vi "openDevice.vi"(8 "error in (no error)":errorcluster, 10 "deviceName":string, 11 "AtomChipHWC in":refnum<class "AtomChipHWC.lvclass">) -> (0 "error out":errorcluster, 3 "AtomChipHWC out":refnum<class "AtomChipHWC.lvclass">)   [LabVIEW 2009, in "Hardware.lvlib" / "HWControllers.lvlib" / "AtomChipHWC.lvclass"]
doc: "Opens a device."
uses:
  AtomChipHWC.lvclass
  IntegrationManagement/CameraManager.lvclass
  AtomChipHWC.lvclass/AtomChipHWC.ctl
  HWController.lvclass
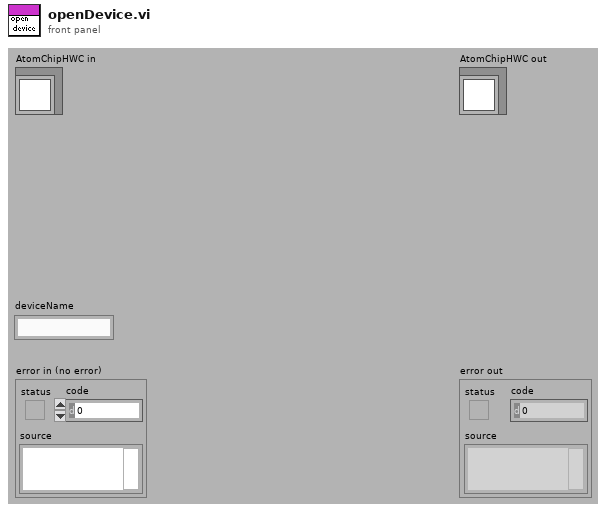
[diagram p1: front panel]
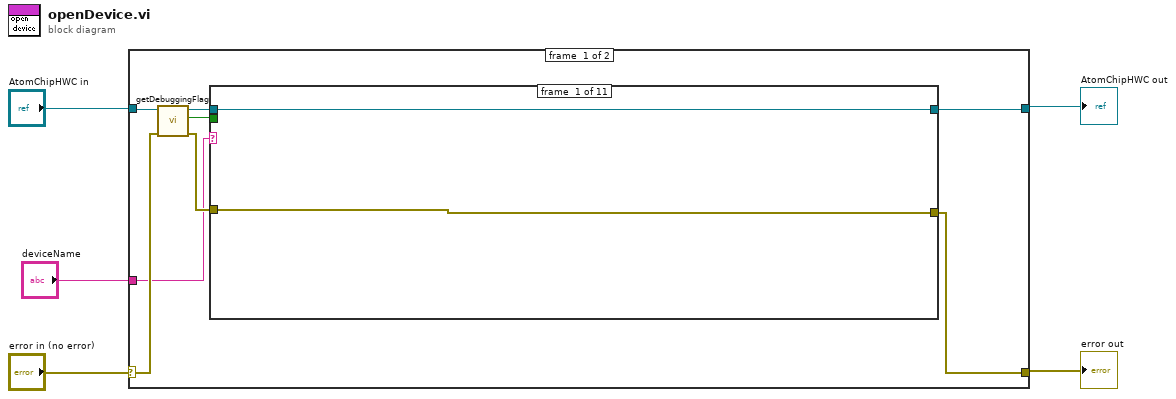
[diagram p0: block diagram]
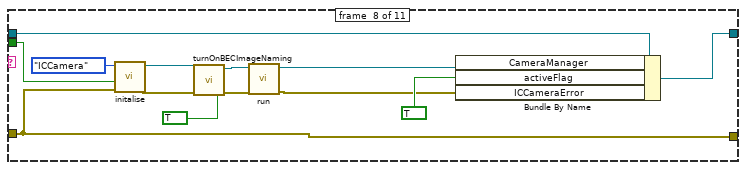
[diagram p8: hidden frame]
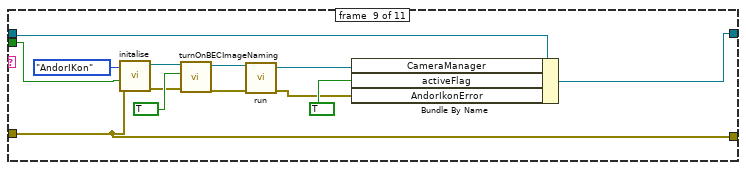
[diagram p9: hidden frame]
diagram:
  n1 = case shown="No Error" "error in (no error)" {
    selector: "error in (no error)" -> [w9 w59]
    tunnel: [w6 w59] -> w4
    tunnel: [w7 w58] -> w2
    tunnel: "AtomChipHWC in" -> [w13 w58]
    tunnel: "deviceName" -> [w8 _]
    frame #0 {
      n2 = call "getDebuggingFlag.vi"("error in (no error)"=w9, "HWController.lvclass in"=w13) -> ("error out"=w10:errorcluster, "debuggingFlag"=w11:bool, "HWController.lvclass out"=w12:refnum<class "AtomChipHWC.lvclass">)  [unwired: 7 in]
      n3 = case shown="\"Dio64\"" w8 {
        tunnel: w12 -> [w15 w17 w19 w21 w22 w25 w27 w38 w51 w55 w57]
        tunnel: [w15 w17 w19 w21 w22 w25 w27 w39 w52 w55 w57] -> w7
        tunnel: w10 -> [w14 w16 w18 w20 w23 w24 w26 w28 w42 w54 w56]
        tunnel: [w14 w16 w18 w20 w23 w24 w26 w28 w42 w54 w56] -> w6
        tunnel: w11 -> [_ _ _ _ _ _ _ w37 w43 _ _]
        frame #0 {
        }
        frame #1 {
        }
        frame #2 {
        }
        frame #3 {
        }
        frame #4 {
        }
        frame #5 {
        }
        frame #6 {
        }
        frame #7 {
          n4 = call "initalise.vi"("error in (no error)"=w28, "Hardware Connected?"=w37, "Camera"=enum16{"AndorIKon", "ICCamera"}."ICCamera") -> ("error out"=w34:errorcluster, "CameraManager out"=w33:refnum<class "CameraManager.lvclass">)  [unwired: 7 in]
          n5 = call "turnOnBECImageNaming.vi"("error in (no error)"=w34, "ImageRenaming"=TRUE, "CameraManager in"=w33) -> ("error out"=w31:errorcluster, "CameraManager out"=w32:refnum<class "CameraManager.lvclass">)  [unwired: 7 in]
          n6 = call-dynamic "run.vi"("error in (no error)"=w31, "CameraManager in"=w32) -> ("error out"=w29:errorcluster, "CameraManager out"=w35:refnum<class "CameraManager.lvclass">)  [unwired: 8 in]
          n7 = Bundle By Name(cluster=w38, "CameraManager"=w35, "activeFlag"=TRUE, "ICCameraError"=w29) -> (w39:refnum<class "AtomChipHWC.lvclass">)
        }
        frame #8 {
          n8 = call "initalise.vi"("error in (no error)"=w42, "Hardware Connected?"=w43, "Camera"=enum16{"AndorIKon", "ICCamera"}."AndorIKon") -> ("error out"=w47:errorcluster, "CameraManager out"=w46:refnum<class "CameraManager.lvclass">)  [unwired: 7 in]
          n9 = call "turnOnBECImageNaming.vi"("error in (no error)"=w47, "ImageRenaming"=TRUE, "CameraManager in"=w46) -> ("error out"=w44:errorcluster, "CameraManager out"=w45:refnum<class "CameraManager.lvclass">)  [unwired: 7 in]
          n10 = call-dynamic "run.vi"("error in (no error)"=w44, "CameraManager in"=w45) -> ("error out"=w41:errorcluster, "CameraManager out"=w50:refnum<class "CameraManager.lvclass">)  [unwired: 8 in]
          n11 = Bundle By Name(cluster=w51, "CameraManager"=w50, "activeFlag"=TRUE, "AndorIkonError"=w41) -> (w52:refnum<class "AtomChipHWC.lvclass">)
        }
        frame #9 {
        }
        frame #10 {
        }
      }
    }
    frame #1 {
    }
  }
  "error out" <- w4
  "AtomChipHWC out" <- w2
